vi "SaveBGorCali (SubVI).vi"(5 "DataType":enum16{"BG", "Cali"}(ring), 6 "SytemID":string(combo)="UCDMC", 7 "BG path":path, 8 "error in (no error)":errorcluster, 9 "Channel 3":cluster{"2DRawDataIn":dbl[][], "CtrlV":dbl[]}, 10 "Channel 2":cluster{"2DRawDataIn":dbl[][], "CtrlV":dbl[]}, 11 "Channel1":cluster{"2DRawDataIn":dbl[][], "CtrlV":dbl[]}) -> (0 "error out":errorcluster)   [LabVIEW 2021]
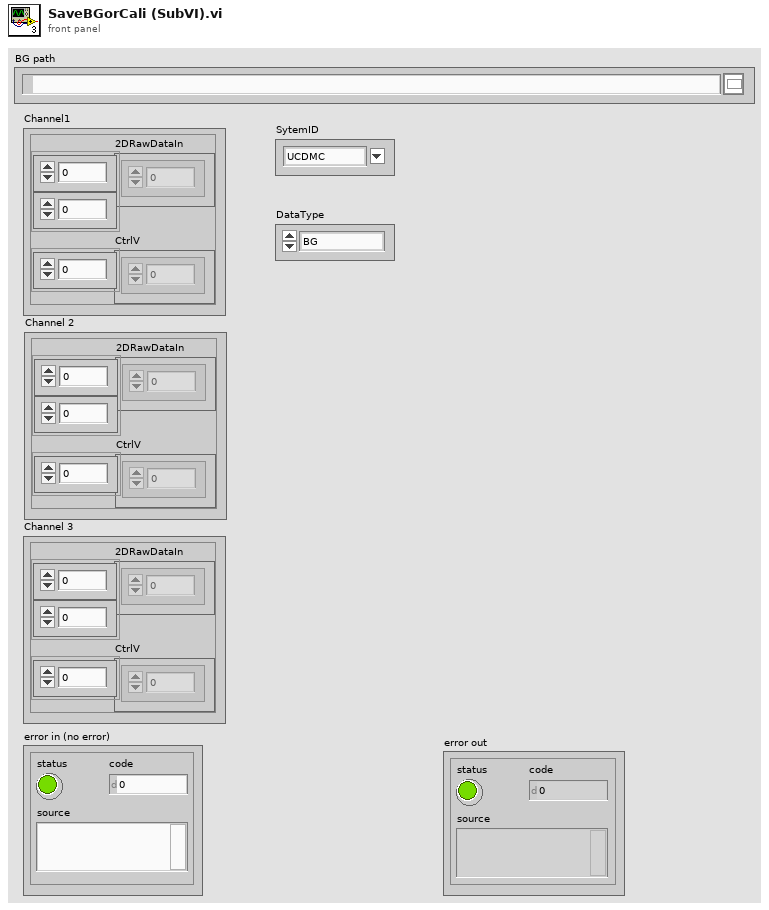
[diagram p1: front panel]
types:
  T1 = enum16{"open", "open or create", "create or replace", "create", "open (read-only)"}
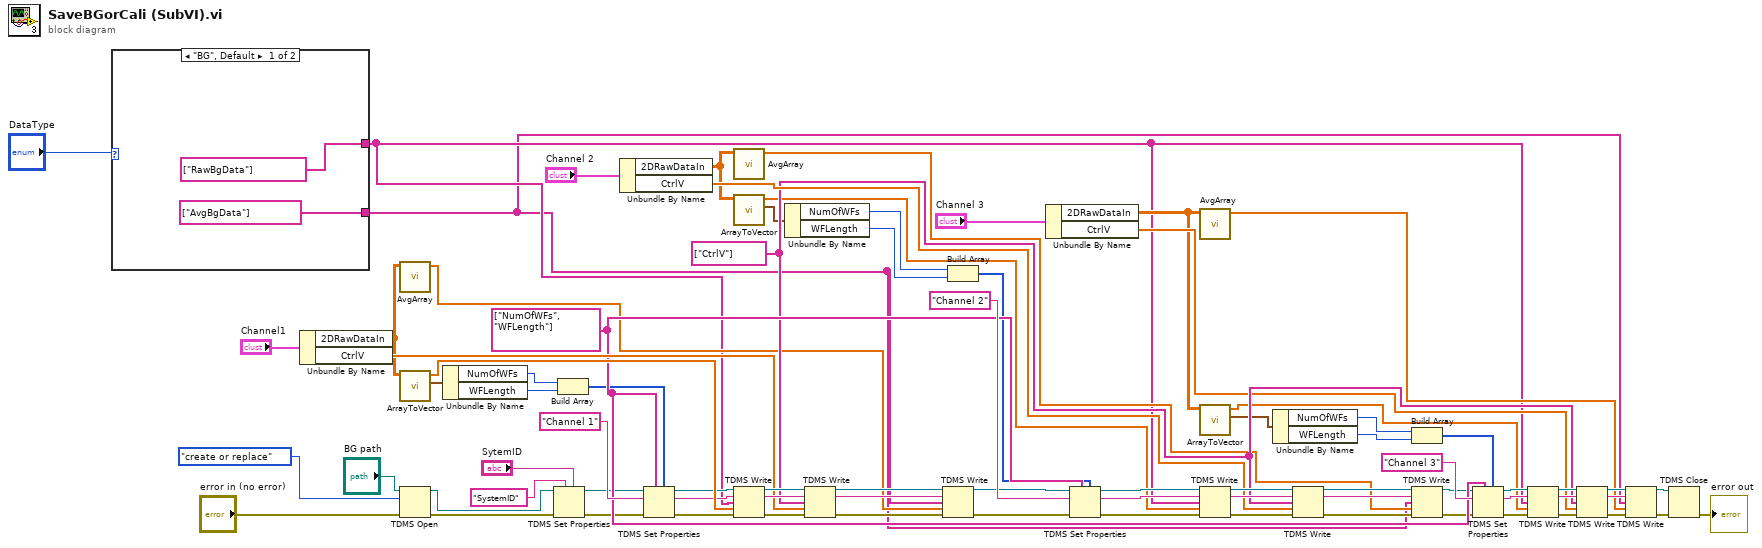
[diagram p0: block diagram]
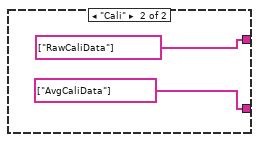
[diagram p2: hidden frame]
diagram:
  w46 = string[] ["CtrlV"] ("channel name(s) in (Untitled)")
  w49 = string[] ["NumOfWFs", "WFLength"] ("property names")
  n1 = case shown="\"BG\", Default" "DataType" {
    tunnel: [string[] ["RawBgData"] ("channel name(s) in (Untitled)") string[] ["RawCaliData"] ("channel name(s) in (Untitled)")] -> w2
    tunnel: [string[] ["AvgBgData"] ("channel name(s) in (Untitled)") string[] ["AvgCaliData"] ("channel name(s) in (Untitled)")] -> w1
    frame "BG", Default {
    }
    frame "Cali" {
    }
  }
  n2 = Unbundle By Name("Channel1") -> ("2DRawDataIn"=w30:dbl[][], "CtrlV"=w67:dbl[])
  n3 = call "AvgArray.vi"("2D array in"=w30) -> ("1D Avg out"=w26:dbl[])  [unwired: 10 in]
  n4 = call "ArrayToVector.vi"("2D WF in"=w30) -> ("WF Dimension"=w44:cluster{"NumOfWFs":i32, "WFLength":i32}, "1D WF out"=w73:dbl[])  [unwired: 9 in]
  n5 = TDMS Open(8:"error in (no error)", 10:T1."create or replace" ("operation (0:open)"), 11:"BG path") -> (0:w8:errorcluster, 3:w9:refnum<k34>)  [unwired: 4 in]
  n6 = Unbundle By Name(w44) -> ("NumOfWFs"=w43:i32, "WFLength"=w42:i32)
  n7 = TDMS Set Properties(5:"SytemID", 7:"SystemID" ("group name in (Untitled)"), 8:w8, 11:w9) -> (0:w6:errorcluster, 3:w7:refnum<k34>)  [unwired: 2 in, 2 out]
  n8 = Build Array(w43, w42) -> (w41:i32[])
  n9 = Unbundle By Name("Channel 2") -> ("2DRawDataIn"=w18:dbl[][], "CtrlV"=w56:dbl[])
  n10 = TDMS Set Properties(5:w41, 7:w49, 8:w6, 10:"Channel 1" ("group name in (Untitled)"), 11:w7) -> (0:w71:errorcluster, 2:w62:string, 3:w72:refnum<k34>)  [unwired: 1 in, 1 out]
  n11 = call "AvgArray.vi"("2D array in"=w18) -> ("1D Avg out"=w17:dbl[])  [unwired: 10 in]
  n12 = call "ArrayToVector.vi"("2D WF in"=w18) -> ("WF Dimension"=w39:cluster{"NumOfWFs":i32, "WFLength":i32}, "1D WF out"=w40:dbl[])  [unwired: 9 in]
  n13 = TDMS Write(0:w72, 5:w62, 7:w2, 9:w73, 11:w71) -> (4:w69:refnum<k34>, 6:w70:string, 15:w68:errorcluster)  [unwired: 1 in, 1 out]
  n14 = Unbundle By Name(w39) -> ("NumOfWFs"=w38:i32, "WFLength"=w37:i32)
  n15 = TDMS Write(0:w69, 5:w70, 7:w46, 9:w67, 11:w68) -> (4:w29:refnum<k34>, 6:w27:string, 15:w28:errorcluster)  [unwired: 1 in, 1 out]
  n16 = TDMS Write(0:w29, 5:w27, 7:w1, 9:w26, 11:w28) -> (4:w25:refnum<k34>, 15:w24:errorcluster)  [unwired: 1 in, 2 out]
  n17 = Build Array(w38, w37) -> (w36:i32[])
  n18 = Unbundle By Name("Channel 3") -> ("2DRawDataIn"=w16:dbl[][], "CtrlV"=w45:dbl[])
  n19 = TDMS Set Properties(5:w36, 7:w49, 8:w24, 10:"Channel 2" ("group name in (Untitled)"), 11:w25) -> (0:w60:errorcluster, 2:w61:string, 3:w64:refnum<k34>)  [unwired: 1 in, 1 out]
  n20 = call "AvgArray.vi"("2D array in"=w16) -> ("1D Avg out"=w13:dbl[])  [unwired: 10 in]
  n21 = call "ArrayToVector.vi"("2D WF in"=w16) -> ("WF Dimension"=w34:cluster{"NumOfWFs":i32, "WFLength":i32}, "1D WF out"=w35:dbl[])  [unwired: 9 in]
  n22 = TDMS Write(0:w64, 5:w61, 7:w2, 9:w40, 11:w60) -> (4:w59:refnum<k34>, 6:w57:string, 15:w58:errorcluster)  [unwired: 1 in, 1 out]
  n23 = Unbundle By Name(w34) -> ("NumOfWFs"=w33:i32, "WFLength"=w32:i32)
  n24 = TDMS Write(0:w59, 5:w57, 7:w46, 9:w56, 11:w58) -> (4:w23:refnum<k34>, 6:w22:string, 15:w21:errorcluster)  [unwired: 1 in, 1 out]
  n25 = Build Array(w33, w32) -> (w31:i32[])
  n26 = TDMS Write(0:w23, 5:w22, 7:w1, 9:w17, 11:w21) -> (4:w20:refnum<k34>, 15:w19:errorcluster)  [unwired: 1 in, 2 out]
  n27 = TDMS Set Properties(5:w31, 7:w49, 8:w19, 10:"Channel 3" ("group name in (Untitled)"), 11:w20) -> (0:w53:errorcluster, 2:w48:string, 3:w54:refnum<k34>)  [unwired: 1 in, 1 out]
  n28 = TDMS Write(0:w54, 5:w48, 7:w2, 9:w35, 11:w53) -> (4:w52:refnum<k34>, 6:w47:string, 15:w51:errorcluster)  [unwired: 1 in, 1 out]
  n29 = TDMS Write(0:w52, 5:w47, 7:w46, 9:w45, 11:w51) -> (4:w15:refnum<k34>, 6:w14:string, 15:w12:errorcluster)  [unwired: 1 in, 1 out]
  n30 = TDMS Write(0:w15, 5:w14, 7:w1, 9:w13, 11:w12) -> (4:w11:refnum<k34>, 15:w10:errorcluster)  [unwired: 1 in, 2 out]
  n31 = TDMS Close(8:w10, 11:w11) -> (0:→"error out":errorcluster)  [unwired: 1 out]
